vi "SubGoal Loop.vi"() -> ()   [LabVIEW 2011]
uses:
  <vilib>/Platform/TimedLoop/XDataNode/timing_clust.ctl
  <vilib>/Platform/TimedLoop/XDataNode/nitl_modes.ctl
  <vilib>/Platform/TimedLoop/XDataNode/wakeup.ctl
  <vilib>/Analysis/coordinate.llb/Angle Units.ctl
  <vilib>/Analysis/coordinate.llb/Angle Range (Degree).ctl
  <vilib>/Analysis/coordinate.llb/Wrap Angle (scalar).vi
  Robot Parameters/Robot Parameters.vi
  <vilib>/Platform/TimedLoop/XDataNode/XDataNode.xnode
  <vilib>/Platform/TimedLoop/XDataNode/XDNodeRunTimeDep.lvlib
  <vilib>/Analysis/NI_AAL_Angle.lvlib
panel:
  out "SubGoal":T1
  out "GPS Data":T1
  out "angle out":dbl
  out "Target Distance":dbl
  out "x < y?":bool
  in  "stop?":bool
  out "error out":errorcluster
  in  "error in":errorcluster
  in  "GPS Waypoint CSV Path":path=path "C:/Users/Moxom/Dropbox/RHRT LabVIEW/Robot Prodcution Code/Sprint 4/Working Code 2/GPS/Waypoints.csv"
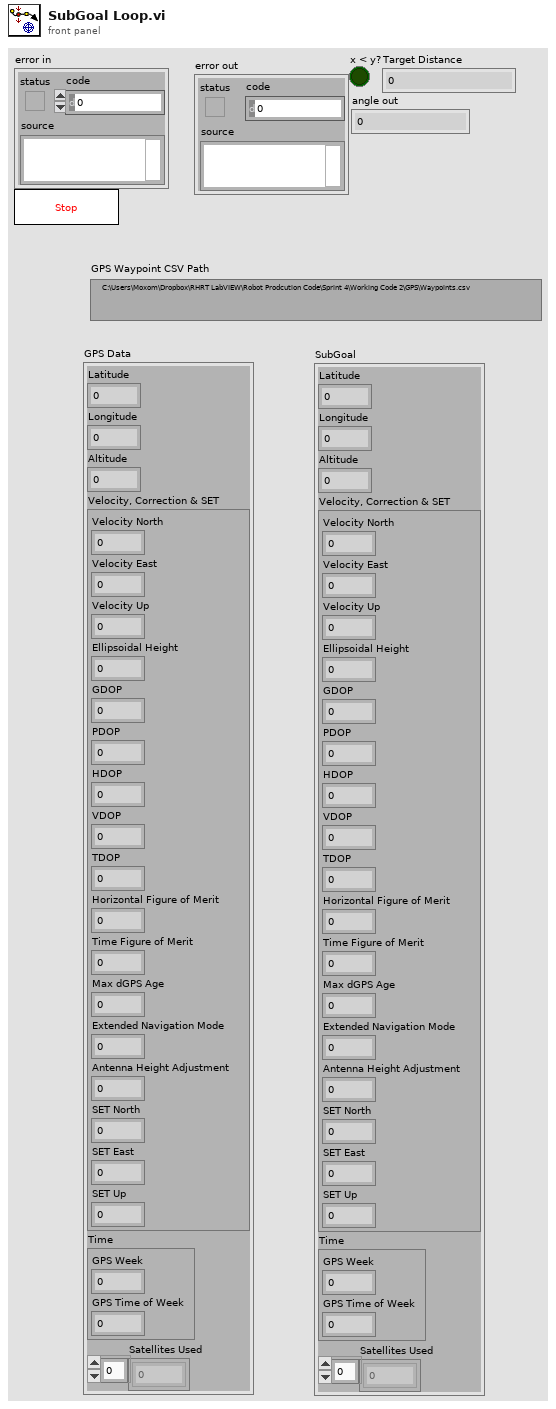
[diagram p1: front panel]
types:
  T1 = cluster{"Latitude":dbl, "Longitude":dbl, "Altitude":dbl, "Velocity, Correction & SET":cluster{"Velocity North":dbl, "Velocity East":dbl, "Velocity Up":dbl, "Ellipsoidal Height":dbl, "GDOP":sgl, "PDOP":sgl, "HDOP":sgl, "VDOP":sgl, "TDOP":sgl, "Horizontal Figure of Merit":u8, "Time Figure of Merit":u8, "Max dGPS Age":sgl, "Extended Navigation Mode":u8, "Antenna Height Adjustment ":dbl, "SET North":i32, "SET East":i32, "SET Up":i32}, "Time":cluster{"GPS Week":u16, "GPS Time of Week":sgl}, "Satellites Used":i32[]}
  T2 = cluster{"Latitude":dbl, "Longitude":dbl, "Altitude":dbl, "Velocity, Correction & SET":cluster{"Velocity North":dbl, "Velocity East":dbl, "Velocity Up":dbl, "Ellipsoidal Height":dbl, "GDOP":sgl, "PDOP":sgl, "HDOP":sgl, "VDOP":sgl, "TDOP":sgl, "Horizontal Figure of Merit":u8, "Time Figure of Merit":u8, "Max dGPS Age":sgl, "Extended Navigation Mode":u8, "Antenna Height Adjustment ":dbl, "SET North":i32, "SET East":i32, "SET Up":i32}, "Time":cluster{"GPS Week":u16, "GPS Time of Week":sgl}, "Satellites Used":i32[]}[]
  T3 = typedef "XDNodeRunTimeDep.lvlib/timing_clust.ctl" = cluster{"Expected End [f-1]":u64, "Actual End [f-1]":u64, "Finished Late? [f-1]":bool, "Expected End [i-1]":u64, "Actual End [i-1]":u64, "Finished Late? [i-1]":bool, "Expected Start [i]":u64, "Actual Start [i]":u64, "Expected Start [f]":u64, "Actual Start [f]":u64, "Source Name":string, "Structure Name":string, "Period":i64, "Deadline":i64, "Offset":i64, "Start":i64, "Priority":i32, "Timeout":i32, "Mode":T4, "Wakeup Reason":T5, "Error":errorcluster, "Source Type":string, "Secondary Source Type":string, "Global End Time":u64, "Global Start Time":u64, "Frame Duration":u64, "Iteration Duration":u64, "Assigned CPU":i32, "I/O Scan Engine Mode":u32}
  T4 = typedef "XDNodeRunTimeDep.lvlib/nitl_modes.ctl" = enum32{"No Change", "Process missed periods, maintain original phase", "Discard missed periods, maintain original phase", "Process missed periods, ignore original phase", "Discard missed periods, ignore original phase"}
  T5 = typedef "XDNodeRunTimeDep.lvlib/wakeup.ctl" = enum32{"Normal", "Aborted", "Asynchronous wakeup", "Timing source error", "Timed loop error", "Timeout"}
  T6 = enum16{"Idle", "Wiimote", "Joypad", "IGVC", "Avoide Objects", "Avoide Lines", "Path Planning", "Heading", "Waypoint"}
  T7 = typedef "NI_AAL_Angle.lvlib/Angle Units.ctl" = i32
  T8 = typedef "NI_AAL_Angle.lvlib/Angle Range (Degree).ctl" = u16
  T9 = cluster{"Position":cluster{"Roll":dbl, "Pitch":dbl, "Yaw":dbl}, "Orientation Matrix":dbl[][], "Magnetic Field":cluster{"Z-Axis Magnetic Field":dbl, "Y-Axis Magnetic Field":dbl, "X-Axis Magnetic Field":dbl}, "Acceleration":cluster{"Z-Axis Acceleration":dbl, "Y-Axis Acceleration":dbl, "X-Axis Acceleration":dbl}, "Angular Rate":cluster{"X-Axis Angular Rate":dbl, "Y-Axis Angular Rate":dbl, "Z-Axis Angular Rate":dbl}, "Quaternion":dbl[]}
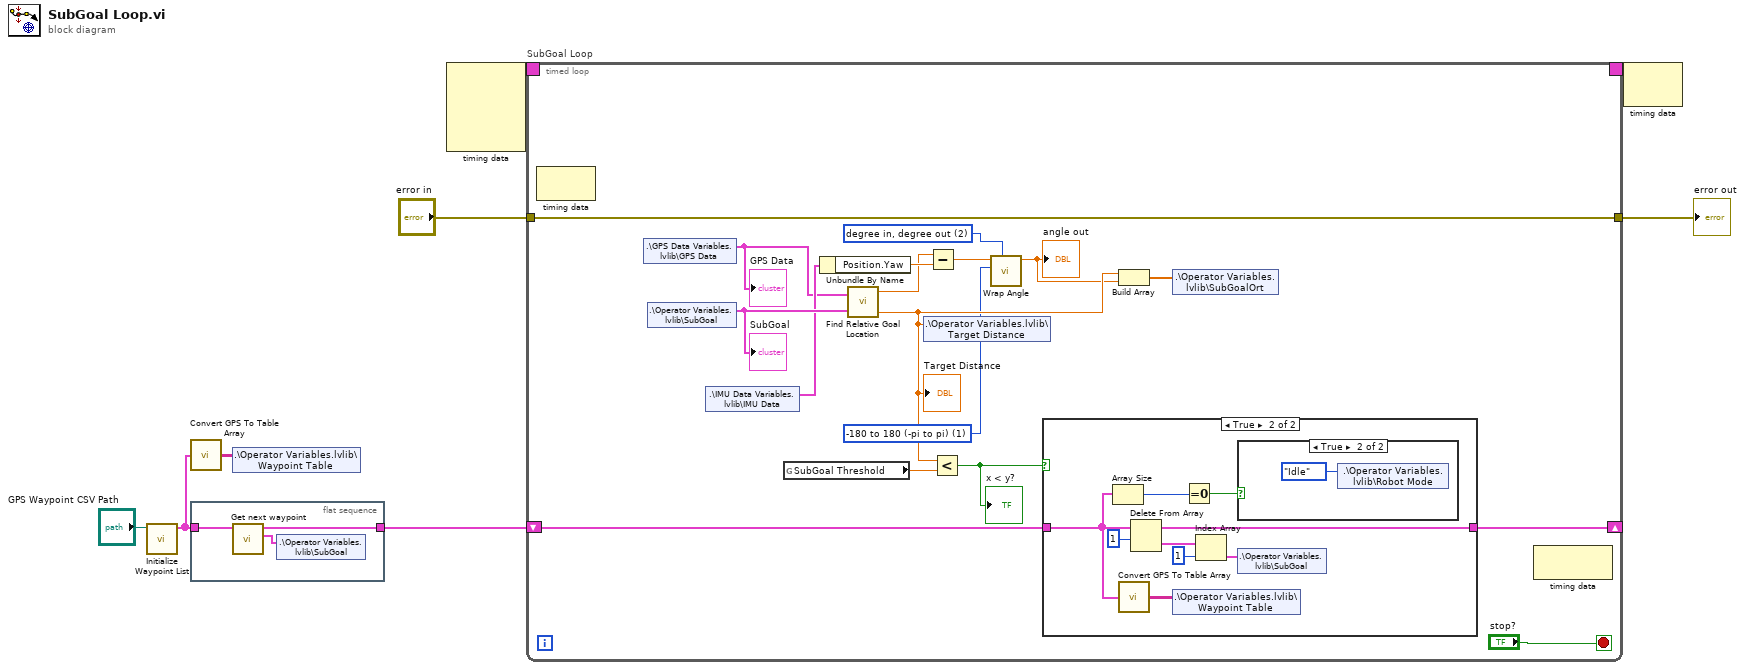
[diagram p0: block diagram]
diagram:
  n1 = call "Initialize Waypoint List.vi"("GPS Waypoint CSV Path"="GPS Waypoint CSV Path") -> ("Waypoint Array"=w2:T2)  [unwired: 10 in]
  n2 = call "Convert GPS To Table Array.vi"("Waypoint Array In"=w2) -> ("Lat/Long Array Out"=w1:string[][])
  n3 = flat-sequence {
    tunnel: w2 -> [w11]
    tunnel: [w10] -> w5
    frame #0 {
      n4 = call "Get next waypoint.vi"("Waypoint Array In"=w11) -> ("Next Waypoint"=w9:T1, "Waypoint Array Out"=w10:T2)  [unwired: 8 in, 1 out]
      n5 = shared-variable ".\\Operator Variables.lvlib\\SubGoal"(w9) -> ()  [unwired: 1 in, 1 out]
    }
  }
  n6 = shared-variable ".\\Operator Variables.lvlib\\Waypoint Table"(w1) -> ()  [unwired: 1 in, 1 out]
  n7 = node-c288() -> (w8:T3)  [unwired: 4 in]
  n8 = timed-loop "SubGoal Loop" {
    timing: w8 -> [_]
    timing-out: [_] -> w7
    tunnel: "error in" -> [w28]
    tunnel: [w28] -> w3
    shift-right: [w25] -> _
    shift-left: w5 -> [w26]
    stop <- "stop?" stop-if-true
    w14 = T7 2 items=["radian in, radian out", "radian in, degree out", "degree in, degree out", "degree in, radian out"] ("angle units")
    w15 = T8 1 items=["none", "-180 to 180 (-pi to pi)", "0 to 360 (0 to 2pi)"] ("angle range")
    n9 = node-c288() -> ()  [unwired: 1 in, 1 out]
    n10 = shared-variable ".\\GPS Data Variables.lvlib\\GPS Data"() -> (w16:T1)  [unwired: 1 in, 1 out]
    "GPS Data" <- w16
    n11 = shared-variable ".\\Operator Variables.lvlib\\SubGoal"() -> (w20:T1)  [unwired: 1 in, 1 out]
    "SubGoal" <- w20
    n12 = shared-variable ".\\IMU Data Variables.lvlib\\IMU Data"() -> (w17:T9)  [unwired: 1 in, 1 out]
    n13 = global read "Robot Parameters.vi" "SubGoal Threshold"() -> (w23:dbl)
    n14 = Unbundle By Name(w17) -> ("Position.Yaw"=w22:dbl)
    n15 = call "Find Relative Goal Location.vi"("Current Position"=w16, "Goal Position"=w20) -> ("Target Heading (deg)"=w21:dbl, "Target Distance"=w19:dbl)  [unwired: 1 out]
    "Target Distance" <- w19
    n16 = shared-variable ".\\Operator Variables.lvlib\\Target Distance"(w19) -> ()  [unwired: 1 in, 1 out]
    n17 = Subtract(x=w21, y=w22) -> (x-y=w13:dbl)
    n18 = Less?(x=w19, y=w23) -> (x < y?=w27:bool)
    "x < y?" <- w27
    n19 = call-poly <vilib>:"Wrap Angle.vi"("angle units"=w14, "angle range"=w15, "angle in"=w13) -> ("angle out"=w12:dbl)  [unwired: 7 in, 1 out]
    "angle out" <- w12
    n20 = case shown="True" w27 {
      tunnel: w26 -> [w29 w31]
      tunnel: [w29 w36] -> w25
      frame False {
      }
      frame True {
        n21 = Array Size(array=w31) -> (size(s)=w32:i32)
        n22 = call "Convert GPS To Table Array.vi"("Waypoint Array In"=w31) -> ("Lat/Long Array Out"=w38:string[][])
        n23 = Delete From Array(array=w31, length=1) -> (deleted portion=w35:T2, array with subset deleted=w36:T2)  [unwired: 1 in]
        n24 = shared-variable ".\\Operator Variables.lvlib\\Waypoint Table"(w38) -> ()  [unwired: 1 in, 1 out]
        n25 = Equal To 0?(x=w32) -> (x = 0?=w30:bool)
        n26 = Index Array(array=w35, index=1) -> (element=w33:T1)
        n27 = case shown="True" w30 {
          frame False {
          }
          frame True {
            n28 = shared-variable ".\\Operator Variables.lvlib\\Robot Mode"(T6."Idle" ("Robot Mode")) -> ()  [unwired: 1 in, 1 out]
          }
        }
        n29 = shared-variable ".\\Operator Variables.lvlib\\SubGoal"(w33) -> ()  [unwired: 1 in, 1 out]
      }
    }
    n30 = Build Array(w19, w12) -> (w18:dbl[])
    n31 = shared-variable ".\\Operator Variables.lvlib\\SubGoalOrt"(w18) -> ()  [unwired: 1 in, 1 out]
    n32 = node-c288() -> ()  [unwired: 1 in, 1 out]
  }
  "error out" <- w3
  n33 = node-c288(w7) -> ()  [unwired: 1 out]
